vi "Serial_UnEscape.vi"(4 "data":u8[](array[numeric]) format="%.0x") -> (1 "data out":u8[](array[numeric]) format="%.0x")   [LabVIEW 2009, in "Serial.lvlib"]
doc: "Remove escaping from the data:\n0xFE 0xFE sequence in data is replaced by byte 0xFF\n0xFE 0xFD sequence in data is replaced by byte 0xFEs"
uses:
  Serial.lvlib
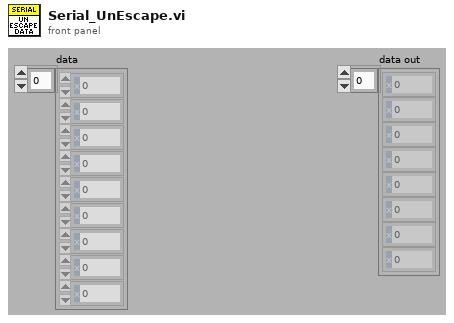
[diagram p1: front panel]
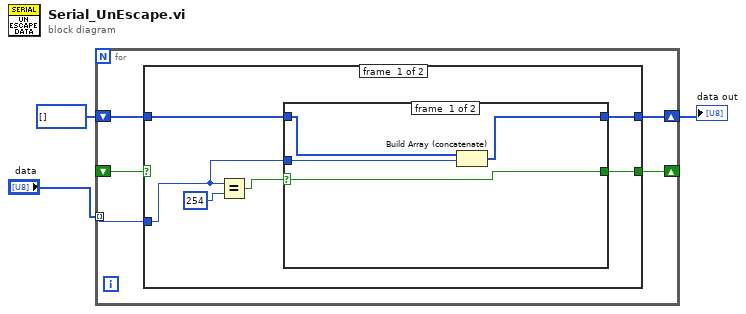
[diagram p0: block diagram]
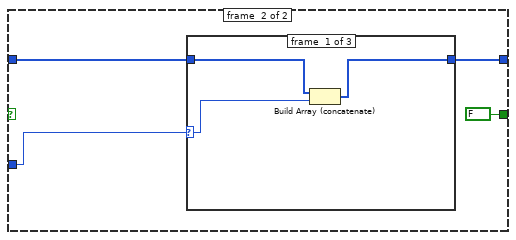
[diagram p3: hidden frame]
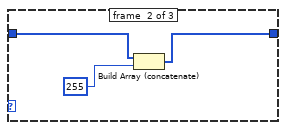
[diagram p4: hidden frame]
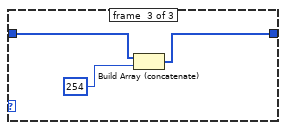
[diagram p5: hidden frame]
diagram:
  n1 = for {
    tunnel: "data" -> [w8] mode=indexing
    shift-right: [w6] -> _
    shift-left: _ -> [w7]
    shift-right: [w5] -> w2
    shift-left: u8[] [] -> [w4]
    n2 = case shown="True" w7 {
      tunnel: w8 -> [w11 w24]
      tunnel: [w12 FALSE] -> w6
      tunnel: [w10 w22] -> w5
      tunnel: w4 -> [w9 w23]
      frame #0 {
        n3 = Equal?(x=w11, y=u8 254) -> (x = y?=w13:bool)
        n4 = case shown="False" w13 {
          selector: w13 -> [w15 w20]
          tunnel: [w15 w20] -> w12
          tunnel: w11 -> [w18 _]
          tunnel: [w17 w19] -> w10
          tunnel: w9 -> [w16 w19]
          frame #0 {
            n5 = Build Array (concatenate)(w16, w18) -> (w17:u8[])
          }
          frame #1 {
          }
        }
      }
      frame #1 {
        n6 = case shown="0, Default" w24 {
          selector: w24 -> [w27 _ _]
          tunnel: w23 -> [w26 w30 w33]
          tunnel: [w25 w28 w31] -> w22
          frame #0 {
            n7 = Build Array (concatenate)(w26, w27) -> (w25:u8[])
          }
          frame #1 {
            n8 = Build Array (concatenate)(w30, u8 255 ("y")) -> (w28:u8[])
          }
          frame #2 {
            n9 = Build Array (concatenate)(w33, u8 254 ("y")) -> (w31:u8[])
          }
        }
      }
    }
  }
  "data out" <- w2
